vi "SECoP-ConvertError.vi"(8 "return is boolean":bool, 9 "return code":i32, 10 "error in (no error)":errorcluster, 11 "DLL path (in)":T1) -> (0 "error out":errorcluster, 3 "DLL path (out)":T1)   [LabVIEW 2023, in "SECoP.lvlib"]
doc: "<b>\"SECoP-ConvertError.vi\"</b> is called from other \"SECoP-*.vi\" to convert a SECoP result code into a human readable error message for LabVIEW's error cluster.\n\n<b>DLL path</b> input and output of cluster from \"SECoP-Initialize.vi\"\n<b>return code</b> SECoP error code to check\n<b>return is boolean</b> check for SECoP error (false) or Unix result (true)"
uses:
  SECoP.lvlib
  Public/SECoP-libraries.ctl
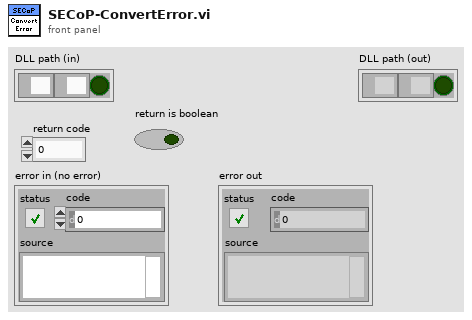
[diagram p1: front panel]
types:
  T1 = typedef "SECoP.lvlib/SECoP-libraries.ctl" = cluster{"serverDLL":path, "variantDLL":path, "cleanup_mode":bool}
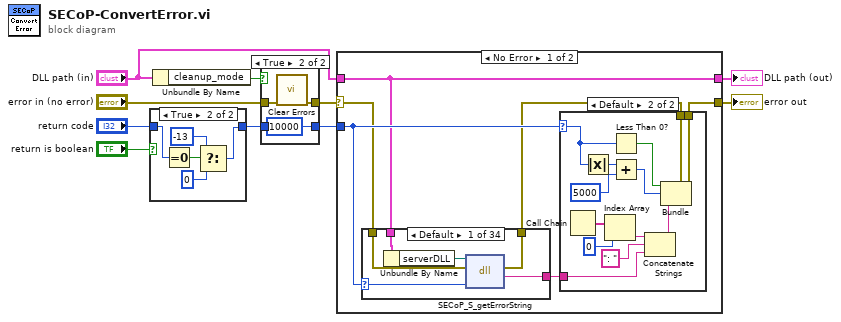
[diagram p0: block diagram]
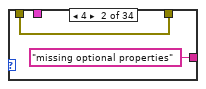
[diagram p4: hidden frame]
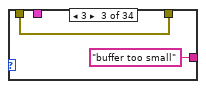
[diagram p5: hidden frame]
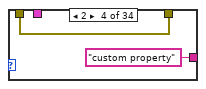
[diagram p6: hidden frame]
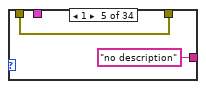
[diagram p7: hidden frame]
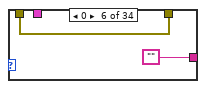
[diagram p8: hidden frame]
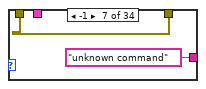
[diagram p9: hidden frame]
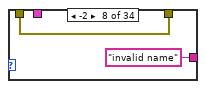
[diagram p10: hidden frame]
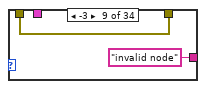
[diagram p11: hidden frame]
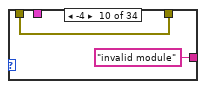
[diagram p12: hidden frame]
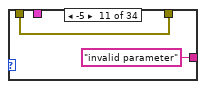
[diagram p13: hidden frame]
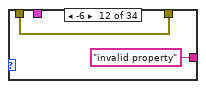
[diagram p14: hidden frame]
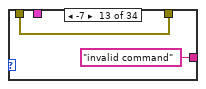
[diagram p15: hidden frame]
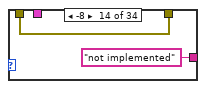
[diagram p16: hidden frame]
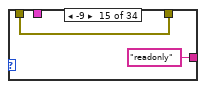
[diagram p17: hidden frame]
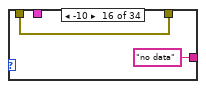
[diagram p18: hidden frame]
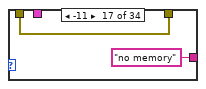
[diagram p19: hidden frame]
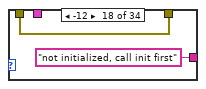
[diagram p20: hidden frame]
diagram:
  n1 = case shown="True" "return is boolean" {
    tunnel: "return code" -> [w11 w16]
    tunnel: [w11 w14] -> w1
    frame False {
    }
    frame True {
      n2 = Equal To 0?(x=w16) -> (x = 0?=w15:bool)
      n3 = Select(t=-13 ("return code"), s=w15, f=0 ("return code")) -> (s? t:f=w14:i32)
    }
  }
  n4 = Unbundle By Name("DLL path (in)") -> ("cleanup_mode"=w7:bool)
  n5 = case shown="True" w7 {
    tunnel: "error in (no error)" -> [w18 w21]
    tunnel: [w18 w20] -> w6
    tunnel: w1 -> [w17 _]
    tunnel: [w17 10000 ("return code")] -> w5
    frame False {
    }
    frame True {
      n6 = call <vilib>:"Clear Errors.vi"("error in (no error)"=w21) -> ("error out"=w20:errorcluster)  [unwired: 5 in, 1 out]
    }
  }
  n7 = case shown="No Error" w6 {
    selector: w6 -> [w23 w114]
    tunnel: w5 -> [w25 _]
    tunnel: "DLL path (in)" -> [w24 w115]
    tunnel: [w24 w115] -> w9
    tunnel: [w27 w114] -> w10
    frame No Error {
      n8 = case shown="Default" w25 {
        selector: w25 -> [w31 _ _ _ _ _ _ _ _ _ _ _ _ _ _ _ _ _ _ _ _ _ _ _ _ _ _ _ _ _ _ _ _ _]
        tunnel: [w30 "missing optional properties" "buffer too small" "custom property" "no description" "" "unknown command" "invalid name" "invalid node" "invalid module" "invalid parameter" "invalid property" "invalid command" "not implemented" "readonly" "no data" "no memory" "not initialized, call init first" "invalid value" "missing mandatory property" "no setter/getter" "no setter" "no getter" "name already in use" "accessible timeout" "wrong bitness" "SECoP-CommandFailed" "SECoP-CommandRunning" "SECoP-CommunicationFailed" "SECoP-IsBusy" "SECoP-IsError" "SECoP-Disabled" "SECoP-SyntaxError" "SECoP-InternalError"] -> w26
        tunnel: w24 -> [w33 _ _ _ _ _ _ _ _ _ _ _ _ _ _ _ _ _ _ _ _ _ _ _ _ _ _ _ _ _ _ _ _ _]
        tunnel: w23 -> [w29 w34 w36 w38 w40 w42 w44 w46 w48 w50 w52 w54 w56 w58 w60 w62 w64 w66 w68 w70 w72 w74 w76 w78 w80 w82 w84 w86 w88 w90 w92 w94 w96 w98]
        tunnel: [w28 w34 w36 w38 w40 w42 w44 w46 w48 w50 w52 w54 w56 w58 w60 w62 w64 w66 w68 w70 w72 w74 w76 w78 w80 w82 w84 w86 w88 w90 w92 w94 w96 w98] -> w22
        frame Default {
          n9 = Unbundle By Name(w33) -> ("serverDLL"=w32:path)
          n10 = dll-call lib="?" fn="SECoP_S_getErrorString"(path in=w32, error in=w29, "iError"=w31) -> (error out=w28:errorcluster, "return type"=w30:string)  [unwired: 2 in, 1 out]
        }
        frame 4 {
        }
        frame 3 {
        }
        frame 2 {
        }
        frame 1 {
        }
        frame 0 {
        }
        frame -1 {
        }
        frame -2 {
        }
        frame -3 {
        }
        frame -4 {
        }
        frame -5 {
        }
        frame -6 {
        }
        frame -7 {
        }
        frame -8 {
        }
        frame -9 {
        }
        frame -10 {
        }
        frame -11 {
        }
        frame -12 {
        }
        frame -13 {
        }
        frame -14 {
        }
        frame -15 {
        }
        frame -16 {
        }
        frame -17 {
        }
        frame -18 {
        }
        frame -19 {
        }
        frame -20 {
        }
        frame -21 {
        }
        frame -22 {
        }
        frame -23 {
        }
        frame -24 {
        }
        frame -25 {
        }
        frame -26 {
        }
        frame -27 {
        }
        frame -28 {
        }
      }
      n11 = case shown="Default" w25 {
        selector: w25 -> [_ w101]
        tunnel: [w100 w111] -> w27
        tunnel: w22 -> [w100 w110]
        tunnel: w26 -> [_ w107]
        frame 0, 10000 {
        }
        frame Default {
          n12 = Call Chain() -> (call chain=w113:string[])
          n13 = Absolute Value(x=w101) -> (abs(x)=w104:i32)
          n14 = Index Array(array=w113, index=0) -> (element=w109:string)
          n15 = Less Than 0?(x=w101) -> (x < 0?=w102:bool)
          n16 = Add(x=w104, y=5000) -> (x+y=w103:i32)
          n17 = Concatenate Strings(w109, ": " ("string"), w107) -> (w106:string)
          n18 = Bundle(cluster=w110, "status"=w102, "code"=w103, "source"=w106) -> (w111:errorcluster)
        }
      }
    }
    frame Error {
    }
  }
  "DLL path (out)" <- w9
  "error out" <- w10
